vi "GOOP_GetClassDynamicVIs.vi"(0 "LvClassIn":refnum<vi>, 5 "error out 2":errorcluster) -> (11 "IsAPropertyDefinitionVI":bool[](array[boolean]), 13 "ConnectorPaneHeight":i32[](array[numeric]), 14 "LvClassOut":refnum<vi>, 15 "ClassName":string, 16 "VINames(without Prefix)":string[](array[string]), 17 "ViPaths":path[](array[path]), 18 "Scope":T1(array[ring]), 19 "error out":errorcluster)   [LabVIEW 2020]
panel:
  # "0 or -1 means Full Icon height\n1 is only one connector terminal height\n  and the header is then removed."
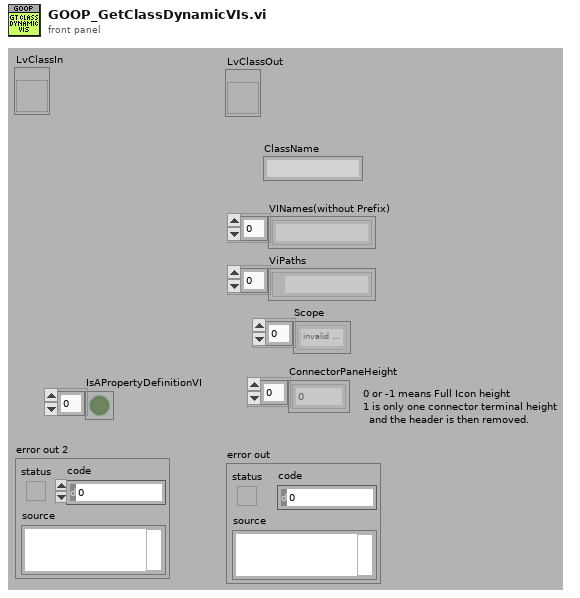
[diagram p1: front panel]
types:
  T1 = enum32{"invalid scope", "public", "private", "protected", "community"}[]
  T2 = enum16{"Invalid Wire Rule", "Required", "Recommended", "Optional", "Dynamic Dispatch"}
  T3 = enum32{"invalid scope", "public", "private", "protected", "community"}
  T4 = enum16{"Invalid Wire Rule", "Required", "Recommended", "Optional", "Dynamic Dispatch"}[]
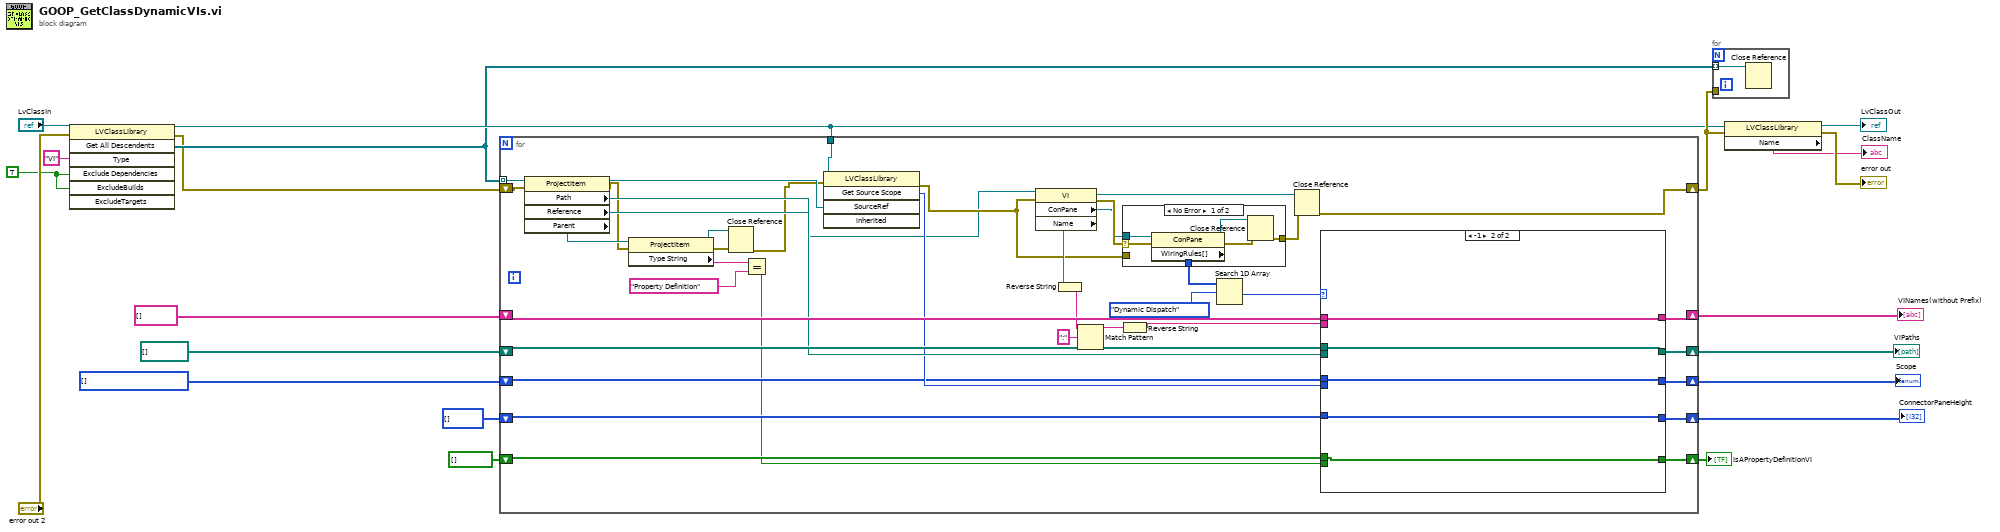
[diagram p0: block diagram]
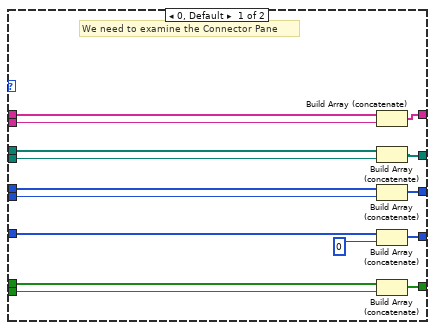
[diagram p3: hidden frame]
diagram:
  w9 = TRUE ("ExcludeDependencies")
  w11 = T1 [] items=["invalid scope", "public", "private", "protected", "community"]
  n1 = invoke class="LVClassLibrary" method="Get All Descendents"(reference="LvClassIn", error in="error out 2", "Type"="VI", "Exclude Dependencies"=w9, "ExcludeBuilds"=w9) -> (reference out=w7:refnum<vi>, error out=w3:errorcluster, "All Descendents"=w6:refnum<vi>[])  [unwired: 2 in, 4 out]
  n2 = for {
    tunnel: w6 -> [w60] mode=indexing
    shift-right: [w52] -> w8
    shift-left: w3 -> [w59]
    shift-right: [w53] -> w21
    shift-left: string[] [] ("Array 2") -> [w54]
    shift-right: [w50] -> w12
    shift-left: path[] [] -> [w49]
    shift-right: [w46] -> w10
    shift-left: w11 -> [w40]
    tunnel: w7 -> [w45]
    shift-right: [w34] -> w5
    shift-left: i32[] [] ("ConnectorPaneHeight") -> [w35]
    shift-right: [w24] -> w1
    shift-left: bool[] [] -> [w23]
    n3 = property class="ProjectItem"(reference=w60, error in=w59) -> (reference out=w44:refnum<vi>, error out=w28:errorcluster, "Path"=w42:path, "Reference"=w39:refnum<vi>, "Parent"=w31:refnum<vi>)
    n4 = property class="ProjectItem"(reference=w31, error in=w28) -> (reference out=w29:refnum<vi>, error out=w30:errorcluster, "Type String"=w26:string)
    n5 = Close Reference(reference=w29, error in (no error)=w30) -> (error out=w27:errorcluster)
    n6 = Equal?(x=w26, y="Property Definition" ("Type String 2")) -> (x = y?=w22:bool)
    n7 = invoke class="LVClassLibrary" method="Get Source Scope"(reference=w45, error in=w27, "SourceRef"=w44) -> (error out=w43:errorcluster, "GetSourceScope"=w41:T3)  [unwired: 2 in, 3 out]
    n8 = property class="VI"(reference=w39, error in=w43) -> (reference out=w32:refnum<vi>, error out=w51:errorcluster, "ConPane"=w33:refnum<vi>, "Name"=w48:string)
    n9 = Reverse String(1:w48) -> (0:w38:string)
    n10 = Match Pattern(string=w38, regular expression=":") -> (before substring=w37:string)  [unwired: 1 in, 3 out]
    n11 = Reverse String(1:w37) -> (0:w36:string)
    n12 = case shown="No Error" w51 {
      selector: w51 -> [w62 _]
      tunnel: w33 -> [w66 _]
      tunnel: [w65 _] -> w58
      tunnel: [w63 w67] -> w56
      tunnel: w43 -> [_ w67]
      frame No Error {
        n13 = property class="ConPane"(reference=w66, error in=w62) -> (reference out=w61:refnum<vi>, error out=w64:errorcluster, "WiringRules[]"=w65:T4)
        n14 = Close Reference(reference=w61, error in (no error)=w64) -> (error out=w63:errorcluster)
      }
      frame Error {
      }
    }
    n15 = Search 1D Array(1D array=w58, element=T2."Dynamic Dispatch") -> (index of element=w55:i32)  [unwired: 1 in]
    n16 = Close Reference(reference=w32, error in (no error)=w56) -> (error out=w52:errorcluster)
    n17 = case shown="-1" w55 {
      tunnel: w54 -> [w82 w87]
      tunnel: [w81 w87] -> w53
      tunnel: w36 -> [w80 _]
      tunnel: [w77 w86] -> w50
      tunnel: w49 -> [w79 w86]
      tunnel: w42 -> [w78 _]
      tunnel: [w76 w85] -> w46
      tunnel: w41 -> [w75 _]
      tunnel: w40 -> [w74 w85]
      tunnel: [w72 w84] -> w34
      tunnel: w35 -> [w73 w84]
      tunnel: [w70 w83] -> w24
      tunnel: w23 -> [w69 w83]
      tunnel: w22 -> [w68 _]
      frame 0, Default {
        # "We need to examine the Connector Pane"
        n18 = Build Array (concatenate)(w82, w80) -> (w81:string[])
        n19 = Build Array (concatenate)(w79, w78) -> (w77:path[])
        n20 = Build Array (concatenate)(w74, w75) -> (w76:T1)
        n21 = Build Array (concatenate)(w73, 0 ("Numeric")) -> (w72:i32[])
        n22 = Build Array (concatenate)(w69, w68) -> (w70:bool[])
      }
      frame -1 {
      }
    }
  }
  "VINames(without Prefix)" <- w21
  "ViPaths" <- w12
  "Scope" <- w10
  "ConnectorPaneHeight" <- w5
  "IsAPropertyDefinitionVI" <- w1
  n23 = for {
    tunnel: w8 -> [_]
    tunnel: w6 -> [w88] mode=indexing
    n24 = Close Reference(reference=w88) -> ()  [unwired: 1 in, 1 out]
  }
  n25 = property class="LVClassLibrary"(reference=w7, error in=w8) -> (reference out=→"LvClassOut":refnum<vi>, error out=→"error out":errorcluster, "Name"=→"ClassName":string)
